vi "Read Operation Condition Register.vi"(8 "error in (no error)":errorcluster, 11 "VISA resource name":refnum<visa-resource-name>) -> (0 "error out":errorcluster, 2 "Data Out":string, 3 "VISA resource name out":refnum<visa-resource-name>)   [LabVIEW 2021, in "Keithley 2450.lvlib"]
doc: "This reads the contents of the Operation Condition Register, which is one of the Operation Event Registers."
uses:
  <instrlib>/Keithley 2450/Keithley 2450.lvlib
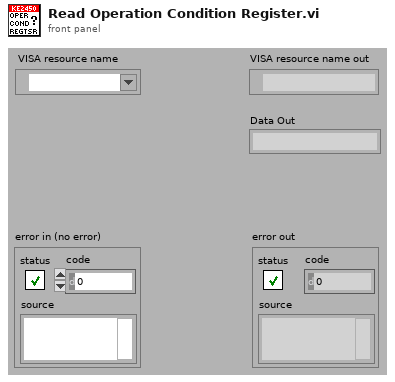
[diagram p1: front panel]
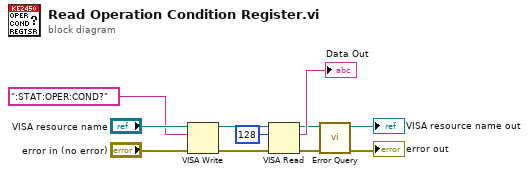
[diagram p0: block diagram]
diagram:
  n1 = VISA Write(VISA resource name="VISA resource name", write buffer=":STAT:OPER:COND?", error in (no error)="error in (no error)") -> (VISA resource name out=w5:refnum<visa-resource-name>, error out=w6:errorcluster)  [unwired: 1 out]
  n2 = VISA Read(VISA resource name=w5, byte count=u32 128, error in (no error)=w6) -> (VISA resource name out=w2:refnum<visa-resource-name>, read buffer=→"Data Out":string, error out=w1:errorcluster)  [unwired: 1 out]
  n3 = call <instrlib>:"Error Query.vi"("error in (no error)"=w1, "VISA resource name"=w2) -> ("error out"=→"error out":errorcluster, "VISA resource name out"=→"VISA resource name out":refnum<visa-resource-name>)  [unwired: 8 out]
